vi "Ctrl-Visibility.vi"(0 "Quick-GUI-Update in":refnum<class "Quick-GUI-Update.lvclass">, 2 "Ctrl-Label":string[](array[string]), 11 "error in (no error)":errorcluster, 13 "Visibility":i32=3) -> (4 "Quick-GUI-Update out":refnum<class "Quick-GUI-Update.lvclass">, 15 "error out":errorcluster)   [LabVIEW 2020, in "Easy GUI Operation.lvlib" / "Quick-GUI-Update.lvclass"]
doc: "<b>Visibility</b>\n1---><b>Show</b> Control's based on the given <b>Ctrl-Label</b> input.\n2---><b>Hide</b> Controls based ont he given <b>Ctrl-Label</b> input.\n3---><b>Show all</b> the control's in the Front Panel."
uses:
  Quick-GUI-Update.lvclass
  Quick-GUI-Update.lvclass/Quick-GUI-Update.ctl
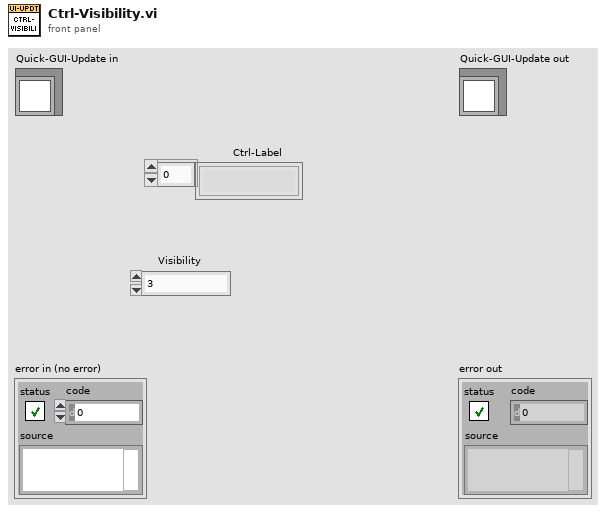
[diagram p1: front panel]
types:
  T1 = map{string, set{cluster{"Ctrl-Ref":refnum<vi>, "Ctrl Index":i32, "Class-Name":string, "Class ID":u32}}}
  T2 = set{cluster{"Ctrl-Ref":refnum<vi>, "Ctrl Index":i32, "Class-Name":string, "Class ID":u32}}
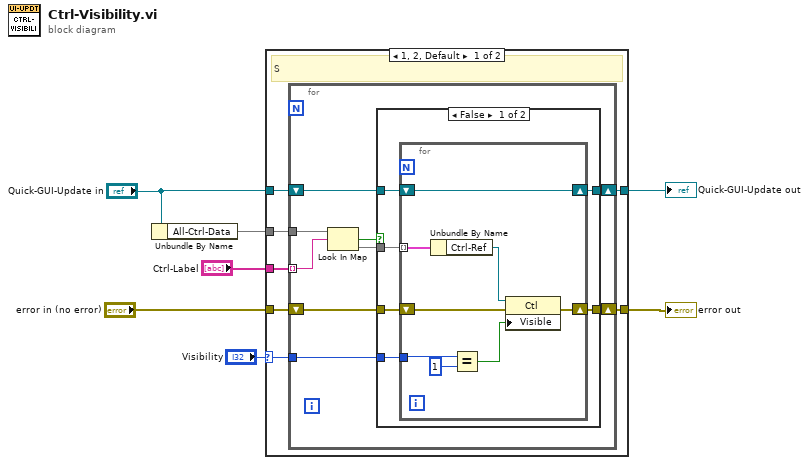
[diagram p0: block diagram]
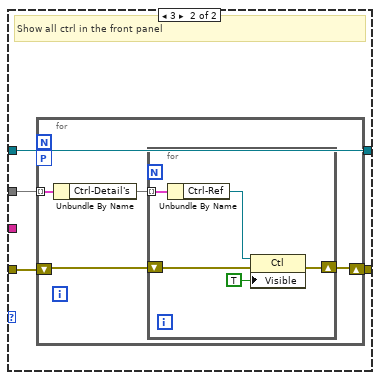
[diagram p3: hidden frame]
diagram:
  n1 = Unbundle By Name("Quick-GUI-Update in") -> ("All-Ctrl-Data"=w1:T1)
  n2 = case shown="1, 2, Default" "Visibility" {
    selector: "Visibility" -> [w13 _]
    tunnel: "Ctrl-Label" -> [w14 _]
    tunnel: "error in (no error)" -> [w12 w43]
    tunnel: "Quick-GUI-Update in" -> [w11 w40]
    tunnel: [w10 w40] -> w4
    tunnel: [w9 w42] -> w6
    tunnel: w1 -> [w8 w41]
    frame 1, 2, Default {
      # "S"
      n3 = for {
        tunnel: w14 -> [w17] mode=indexing
        tunnel: w13 -> [w22]
        shift-right: [w23] -> w9
        shift-left: w12 -> [w21]
        shift-right: [w19] -> w10
        shift-left: w11 -> [w20]
        tunnel: w8 -> [w18]
        n4 = Look In Map(map=w18, key=w17) -> (key not found?=w16:bool, value=w15:T2)  [unwired: 1 in]
        n5 = case shown="False" w16 {
          tunnel: [w29 w38] -> w23
          tunnel: w22 -> [w28 _]
          tunnel: w21 -> [w27 w38]
          tunnel: w20 -> [w26 w39]
          tunnel: [w25 w39] -> w19
          tunnel: w15 -> [w24 _]
          frame False {
            n6 = for {
              tunnel: w28 -> [w32]
              shift-right: [w33] -> w29
              shift-left: w27 -> [w34]
              shift-right: [w37] -> w25
              shift-left: w26 -> [w37]
              tunnel: w24 -> [w36] mode=indexing
              n7 = Unbundle By Name(w36) -> ("Ctrl-Ref"=w35:refnum<vi>)
              n8 = Equal?(x=w32, y=1) -> (x = y?=w30:bool)
              n9 = property class="Ctl"(reference=w35, error in=w34, "Visible"=w30) -> (error out=w33:errorcluster)  [unwired: 1 out]
            }
          }
          frame True {
          }
        }
      }
    }
    frame 3 {
      # "Show all ctrl in the front panel"
      n10 = for {
        shift-right: [w45] -> w42
        shift-left: w43 -> [w44]
        tunnel: w41 -> [w47] mode=indexing
        workers-P: _ -> [_]
        n11 = Unbundle By Name(w47) -> ("Ctrl-Detail's"=w46:T2)
        n12 = for {
          tunnel: w46 -> [w52] mode=indexing
          shift-right: [w49] -> w45
          shift-left: w44 -> [w50]
          n13 = Unbundle By Name(w52) -> ("Ctrl-Ref"=w51:refnum<vi>)
          n14 = property class="Ctl"(reference=w51, error in=w50, "Visible"=TRUE) -> (error out=w49:errorcluster)  [unwired: 1 out]
        }
      }
    }
  }
  "error out" <- w6
  "Quick-GUI-Update out" <- w4
